vi "TCP-Send Strings (byte array).vi"(0 "PXI Address":string, 5 "Port":i32, 7 "strings":string[](array[string]), 11 "error in (no error)":errorcluster) -> (8 "result":i32, 15 "error out":errorcluster)   [LabVIEW 2020]
panel:
  in  "timeout (ms)":i32=5000
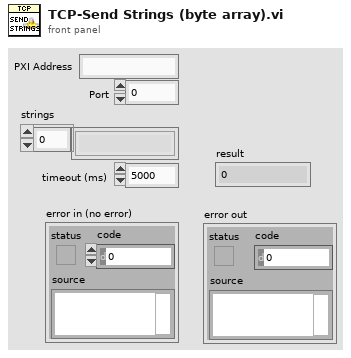
[diagram p1: front panel]
types:
  T1 = enum16{"Standard", "Buffered", "CRLF", "Immediate"}
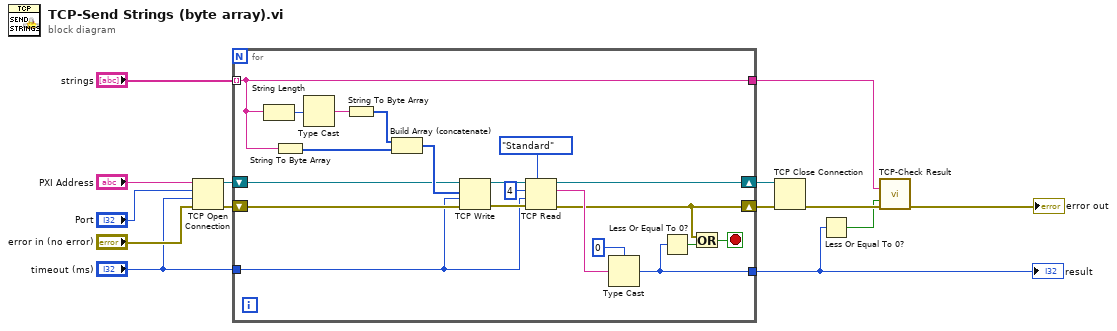
[diagram p0: block diagram]
diagram:
  n1 = TCP Open Connection(address="PXI Address", remote port or service name="Port", timeout ms (60000)="timeout (ms)", error in (no error)="error in (no error)") -> (connection ID=w12:refnum<k5>, error out=w7:errorcluster)  [unwired: 1 in]
  n2 = for {
    tunnel: [w18] -> w10
    tunnel: "timeout (ms)" -> [w23]
    tunnel: "strings" -> [w19] mode=indexing
    shift-right: [w27] -> w8
    shift-left: w12 -> [w32]
    shift-right: [w16] -> w9
    shift-left: w7 -> [w24]
    tunnel: [w19] -> w3
    stop <- w15 stop-if-true
    n3 = String Length(string=w19) -> (length=w22:i32)
    n4 = String To Byte Array(string=w19) -> (unsigned byte array=w34:u8[])
    n5 = Type Cast(x=w22) -> (*(type *) &x=w21:string)  [unwired: 1 in]
    n6 = String To Byte Array(string=w21) -> (unsigned byte array=w20:u8[])
    n7 = Build Array (concatenate)(w20, w34) -> (w33:u8[])
    n8 = TCP Write(connection ID=w32, data in=w33, error in (no error)=w24, 9:w23) -> (connection ID out=w26:refnum<k5>, error out=w25:errorcluster)  [unwired: 1 out]
    n9 = TCP Read(connection ID=w26, bytes to read=4, error in (no error)=w25, 7:T1."Standard" ("mode (standard)"), 9:w23) -> (connection ID out=w27:refnum<k5>, data out=w28:string, error out=w16:errorcluster)
    n10 = Type Cast(type=0, x=w28) -> (*(type *) &x=w18:i32)
    n11 = Less Or Equal To 0?(x=w18) -> (x <= 0?=w17:bool)
    n12 = Or(x=w16, y=w17) -> (x .or. y?=w15:bool)
  }
  "result" <- w10
  n13 = TCP Close Connection(connection ID=w8, error in (no error)=w9) -> (error out=w4:errorcluster)  [unwired: 1 in, 1 out]
  n14 = Less Or Equal To 0?(x=w10) -> (x <= 0?=w2:bool)
  n15 = call "TCP-Check Result.vi"("command"=w3, "invalid response"=w2, "error IO"=w4) -> ("error out"=→"error out":errorcluster)  [unwired: 12 in]
